vi "Initialize Format String.vi"(8 "error in (no error)":errorcluster, 11 "Numeric Data Type in":refnum<class "Numeric Data Type.lvclass">) -> (0 "error out":errorcluster, 3 "Numeric Data Type (dup)":refnum<class "Numeric Data Type.lvclass">)   [LabVIEW 2018, in "Numeric Data Type.lvclass"]
uses:
  Numeric Data Type.lvclass
  Numeric Data Type.lvclass/Numeric Data Type.ctl
  Reference Format String.vi
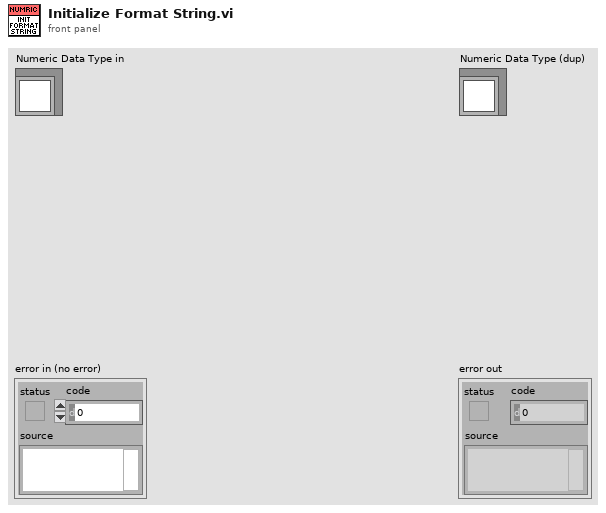
[diagram p1: front panel]
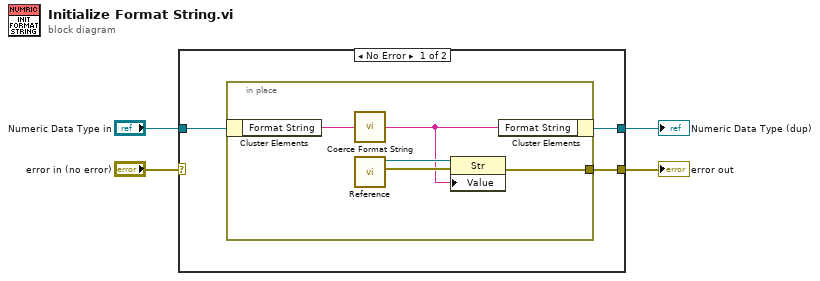
[diagram p0: block diagram]
diagram:
  n1 = case shown="No Error" "error in (no error)" {
    selector: "error in (no error)" -> [_ w14]
    tunnel: [w7 w14] -> w3
    tunnel: [w5 w13] -> w1
    tunnel: "Numeric Data Type in" -> [w6 w13]
    frame No Error {
      n2 = in-place {
        in-place-border: [w10] -> w7
        n3 = in-place-cluster #1(w6) -> ("Format String"=w9:string)
        n4 = call "Coerce Format String.vi"("Format String"=w9) -> ("Coerced String"=w8:string)
        n5 = call-poly "Reference.vi"() -> ("error out"=w11:errorcluster, "Format String"=w12:refnum<vi>)  [unwired: 10 in]
        n6 = property class="Str"(reference=w12, error in=w11, "Value"=w8) -> (error out=w10:errorcluster)  [unwired: 1 out]
        n7 = in-place-cluster #1("Format String"=w8) -> (w5:refnum<class "Numeric Data Type.lvclass">)
      }
    }
    frame Error {
    }
  }
  "error out" <- w3
  "Numeric Data Type (dup)" <- w1
